vi "ConvertToCustomisedXML.vi"(8 "error in":errorcluster, 9 "New Element":refnum<k20>, 10 "DOM document":refnum<k20>, 11 "Path":path) -> (0 "error out":errorcluster, 3 "DOM document out":refnum<k20>)   [LabVIEW 2011]
uses:
  Data.ctl
  Program Files (x86)/National Instruments/LabVIEW 2011/resource/objmgr/DOMUserDefRef.rc
panel:
  out "size(s)":i32
  out "value":T1[](array[typedef])
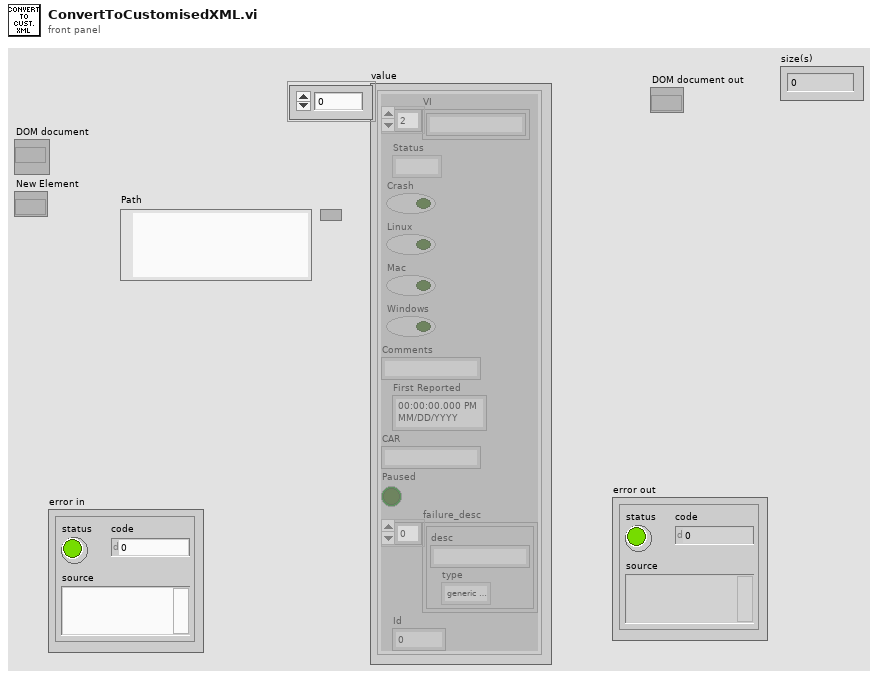
[diagram p1: front panel]
types:
  T1 = typedef "Data.ctl" = cluster{"VI":string[], "Status":enum16{"", "new", "passed", "known"}, "Crash":bool, "Linux":bool, "Mac":bool, "Windows":bool, "Comments":string, "First Reported":timestamp, "CAR":string, "Paused":bool, "failure_desc":cluster{"desc":string, "type":enum32{"generic failure", "boundary case", "precision", "expected error"}}[], "Id":i32}
  T2 = cluster{"desc":string, "type":enum32{"generic failure", "boundary case", "precision", "expected error"}}[]
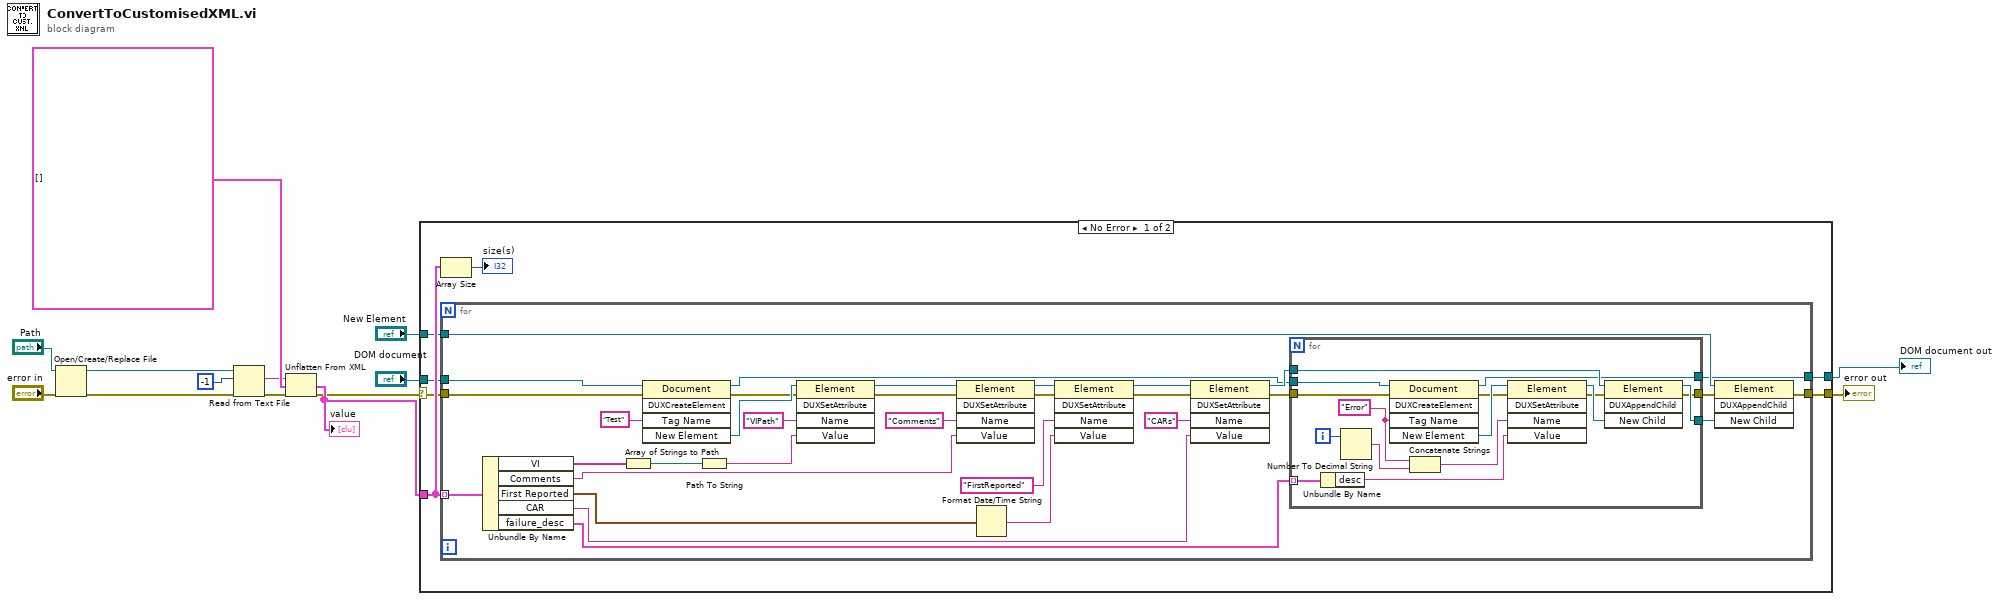
[diagram p0: block diagram]
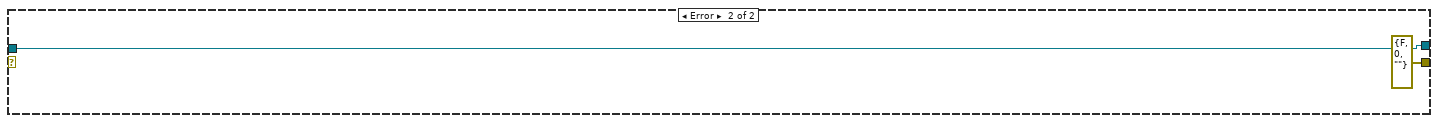
[diagram p2: hidden frame]
diagram:
  n1 = Open/Create/Replace File(file path (use dialog)="Path", error in="error in") -> (refnum out=w10:refnum<file>, error out=w9:errorcluster)  [unwired: 4 in, 1 out]
  n2 = Read from Text File(file (use dialog)=w10, count=-1, error in=w9) -> (text=w12:string, error out=w8:errorcluster)  [unwired: 1 in, 2 out]
  n3 = Unflatten From XML(xml string=w12, type=T1[] [] ("Loaded Data in"), error in (no error)=w8) -> (value=w7:T1[], error out=w1:errorcluster)
  "value" <- w7
  n4 = case shown="No Error" w1 {
    selector: w1 -> [w15 _]
    tunnel: w7 -> [w20 _]
    tunnel: "DOM document" -> [w19 w71]
    tunnel: "New Element" -> [w18 _]
    tunnel: [w17 w71] -> w3
    tunnel: [w16 errorcluster {"status"=FALSE, "code"=0, "source"=""} ("error out")] -> w2
    frame No Error {
      n5 = Array Size(array=w20) -> (size(s)=→"size(s)":i32)
      n6 = for {
        tunnel: w20 -> [w53] mode=indexing
        tunnel: w18 -> [w35]
        tunnel: [w22] -> w17
        tunnel: w15 -> [w33]
        tunnel: [w25] -> w16
        tunnel: w19 -> [w24]
        n7 = Unbundle By Name(w53) -> ("VI"=w49:string[], "Comments"=w45:string, "First Reported"=w43:timestamp, "CAR"=w39:string, "failure_desc"=w36:T2)
        n8 = Array of Strings to Path(0:w49) -> (2:w48:path)  [unwired: 1 in]
        n9 = invoke class="Document" method="DUXCreateElement"(reference=w24, error in=w33, "Tag Name"="Test") -> (reference out=w23:refnum<k20>, error out=w32:errorcluster, "New Element"=w51:refnum<k20>)  [unwired: 2 in, 2 out]
        n10 = Path To String(path=w48) -> (string=w31:string)
        n11 = invoke class="Element" method="DUXSetAttribute"(reference=w51, error in=w32, "Name"="VIPath", "Value"=w31) -> (reference out=w46:refnum<k20>, error out=w30:errorcluster)  [unwired: 1 in, 3 out]
        n12 = invoke class="Element" method="DUXSetAttribute"(reference=w46, error in=w30, "Name"="Comments", "Value"=w45) -> (reference out=w44:refnum<k20>, error out=w29:errorcluster)  [unwired: 1 in, 3 out]
        n13 = Format Date/Time String(seconds (now)=w43) -> (date/time string=w42:string)  [unwired: 2 in]
        n14 = invoke class="Element" method="DUXSetAttribute"(reference=w44, error in=w29, "Name"="FirstReported", "Value"=w42) -> (reference out=w40:refnum<k20>, error out=w28:errorcluster)  [unwired: 1 in, 3 out]
        n15 = invoke class="Element" method="DUXSetAttribute"(reference=w40, error in=w28, "Name"="CARs", "Value"=w39) -> (reference out=w37:refnum<k20>, error out=w27:errorcluster)  [unwired: 1 in, 3 out]
        n16 = for {
          tunnel: w37 -> [w62]
          tunnel: w36 -> [w67] mode=indexing
          tunnel: [w60] -> w34
          tunnel: w27 -> [w59]
          tunnel: [w56] -> w26
          tunnel: w23 -> [w55]
          tunnel: [w54] -> w22
          i -> [w69]
          w63 = "Error" ("string")
          n17 = Unbundle By Name(w67) -> ("desc"=w66:string)
          n18 = Number To Decimal String(number=w69) -> (decimal integer string=w68:string)  [unwired: 1 in]
          n19 = invoke class="Document" method="DUXCreateElement"(reference=w55, error in=w59, "Tag Name"=w63) -> (reference out=w54:refnum<k20>, error out=w58:errorcluster, "New Element"=w65:refnum<k20>)  [unwired: 2 in, 2 out]
          n20 = Concatenate Strings(w63, w68) -> (w64:string)
          n21 = invoke class="Element" method="DUXSetAttribute"(reference=w65, error in=w58, "Name"=w64, "Value"=w66) -> (reference out=w61:refnum<k20>, error out=w57:errorcluster)  [unwired: 1 in, 3 out]
          n22 = invoke class="Element" method="DUXAppendChild"(reference=w62, error in=w57, "New Child"=w61) -> (reference out=w60:refnum<k20>, error out=w56:errorcluster)  [unwired: 1 in, 2 out]
        }
        n23 = invoke class="Element" method="DUXAppendChild"(reference=w35, error in=w26, "New Child"=w34) -> (error out=w25:errorcluster)  [unwired: 1 in, 3 out]
      }
    }
    frame Error {
    }
  }
  "error out" <- w2
  "DOM document out" <- w3
